vi "Read File-group-channel.vi"(8 "error in (no error)":errorcluster, 11 "XY Plot in":refnum<class "XY Plot.lvclass">) -> (0 "error out":errorcluster, 2 "File-group-channel":T1(array[cluster]), 3 "XY Plot out":refnum<class "XY Plot.lvclass">)   [LabVIEW 2016, in "XY Plot.lvclass"]
uses:
  XY Plot.lvclass
  XY Plot.lvclass/XY Plot.ctl
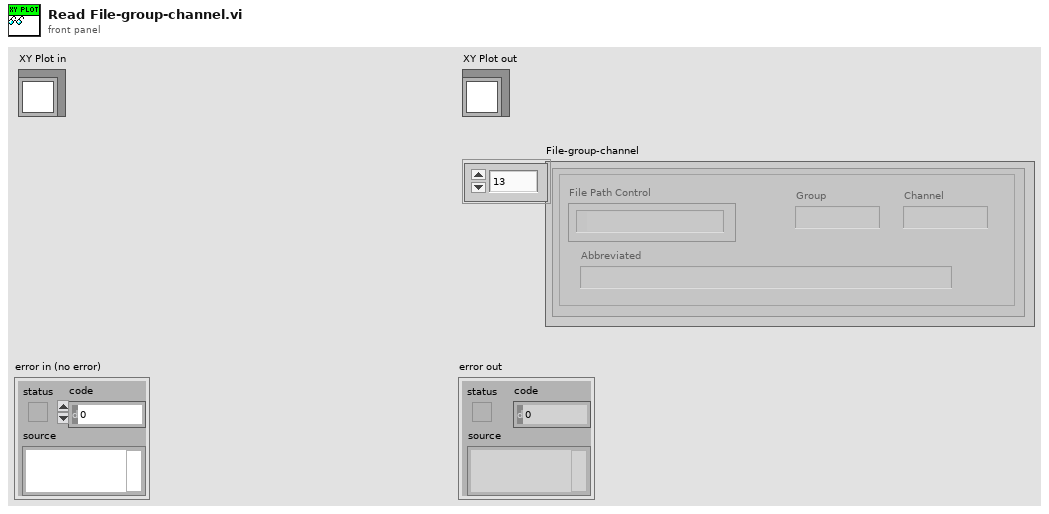
[diagram p1: front panel]
types:
  T1 = cluster{"File Path Control":path, "Group":string, "Channel":string, "Abbreviated":string}[]
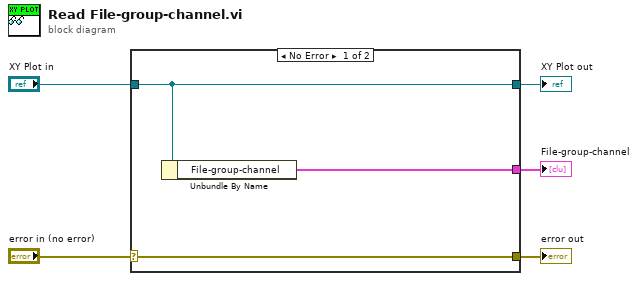
[diagram p0: block diagram]
diagram:
  n1 = case shown="No Error" "error in (no error)" {
    selector: "error in (no error)" -> [w8 w9]
    tunnel: [w8 w9] -> w4
    tunnel: [w7 w10] -> w2
    tunnel: "XY Plot in" -> [w7 w10]
    tunnel: [w6 _] -> w1
    frame No Error {
      n2 = Unbundle By Name(w7) -> ("File-group-channel"=w6:T1)
    }
    frame Error {
    }
  }
  "error out" <- w4
  "XY Plot out" <- w2
  "File-group-channel" <- w1
